vi "Unregister Open Handle.vi"(8 "error in":errorcluster, 10 "handle":T1 format="%02x", 11 "session in":refnum<class "Session.lvclass">) -> (0 "error out":errorcluster, 3 "session out":refnum<class "Session.lvclass">)   [LabVIEW 2020, in "NI_SFTP.lvlib" / "Session.lvclass"]
uses:
  <vilib>/net/SFTP/Session/Session.lvclass
  <vilib>/net/SFTP/Session/Handle.ctl
  <vilib>/net/SFTP/Session/Session.lvclass/Session.ctl
  <vilib>/Utility/error.llb/Error Cluster From Error Code.vi
  <vilib>/ErrorRing/Error Ring.xnode
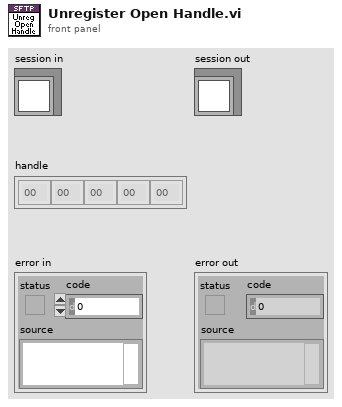
[diagram p1: front panel]
types:
  T1 = typedef "NI_SFTP.lvlib/Session.lvclass/Handle.ctl" = u8[]
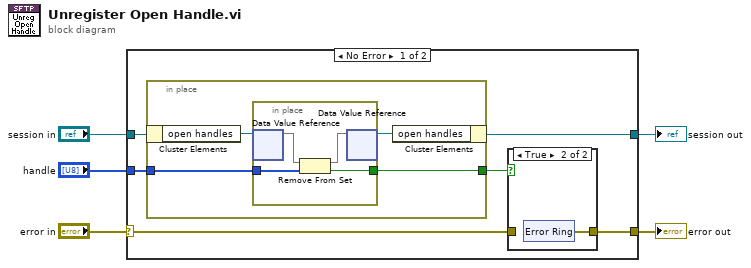
[diagram p0: block diagram]
diagram:
  n1 = case shown="No Error" "error in" {
    selector: "error in" -> [w7 w27]
    tunnel: [w6 w27] -> w1
    tunnel: [w9 w26] -> w2
    tunnel: "session in" -> [w11 w26]
    tunnel: "handle" -> [w10 _]
    frame No Error {
      n2 = in-place {
        in-place-border: w10 -> [w20]
        in-place-border: [w18] -> w8
        n3 = in-place-cluster #1(w11) -> ("open handles"=w21:refnum<data-value>)
        n4 = in-place {
          in-place-border: w20 -> [w24]
          in-place-border: [w22] -> w18
          n5 = in-place-dvr #2(w21) -> (w25:set{T1})  [unwired: 1 out]
          n6 = Remove From Set(10:w24, 11:w25) -> (2:w22:bool, 3:w23:set{T1})
          n7 = in-place-dvr #2(w23) -> (w19:refnum<data-value>)  [unwired: 1 out]
        }
        n8 = in-place-cluster #1("open handles"=w19) -> (w9:refnum<class "Session.lvclass">)
      }
      n9 = case shown="True" w8 {
        tunnel: w7 -> [w12 _]
        tunnel: [w12 w13] -> w6
        frame False {
        }
        frame True {
          n10 = xnode "Error Ring"() -> ("error out"=w13:errorcluster)
        }
      }
    }
    frame Error {
    }
  }
  "error out" <- w1
  "session out" <- w2
